vi "Play.vi"(8 "error in (no error)":errorcluster, 9 "fileName":string, 10 "audioType":string, 11 "MediaAdapter in":refnum<class "MediaAdapter.lvclass">) -> (0 "error out":errorcluster, 3 "MediaAdapter out":refnum<class "MediaAdapter.lvclass">)   [LabVIEW 2017, in "MediaAdapter.lvclass"]
uses:
  MediaAdapter.lvclass
  MediaAdapter.lvclass/MediaAdapter.ctl
  Advanced Media Player/AdvancedMediaPlayer.lvclass
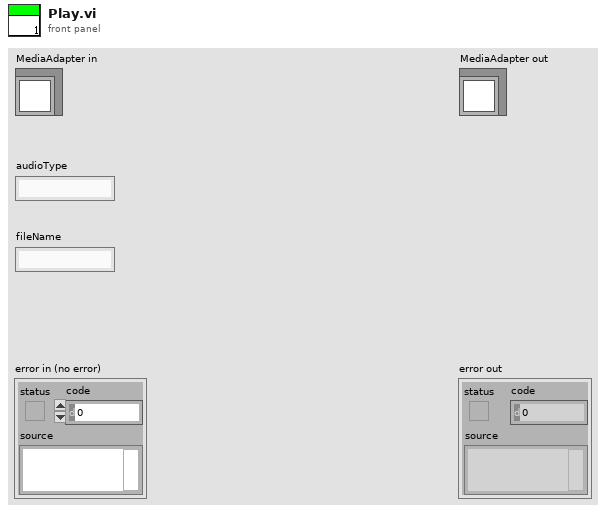
[diagram p1: front panel]
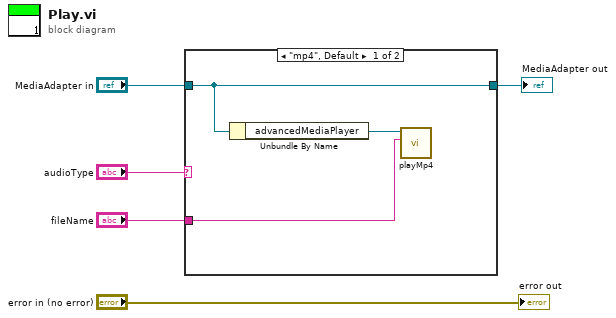
[diagram p0: block diagram]
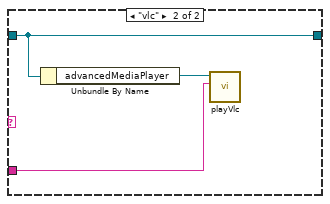
[diagram p2: hidden frame]
diagram:
  n1 = case shown="\"mp4\", Default" "audioType" {
    tunnel: [w8 w11] -> w3
    tunnel: "MediaAdapter in" -> [w8 w11]
    tunnel: "fileName" -> [w6 w9]
    frame "mp4", Default {
      n2 = Unbundle By Name(w8) -> ("advancedMediaPlayer"=w7:refnum<class "AdvancedMediaPlayer.lvclass">)
      n3 = call-dynamic "playMp4.vi"("playMp4"=w6, "AdvancedMediaPlayer in"=w7) -> ()  [unwired: 8 in, 2 out]
    }
    frame "vlc" {
      n4 = Unbundle By Name(w11) -> ("advancedMediaPlayer"=w10:refnum<class "AdvancedMediaPlayer.lvclass">)
      n5 = call-dynamic "playVlc.vi"("playVlc"=w9, "AdvancedMediaPlayer in"=w10) -> ()  [unwired: 8 in, 2 out]
    }
  }
  "MediaAdapter out" <- w3
  "error out" <- "error in (no error)"
